vi "saveGlobalVar-2.vi"() -> ()   [LabVIEW 2019]
uses:
  GlobalVariable1.vi
panel:
  out "Waveform Chart":dbl(graph)
  in  "stop":bool
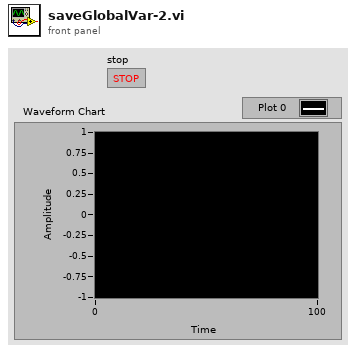
[diagram p1: front panel]
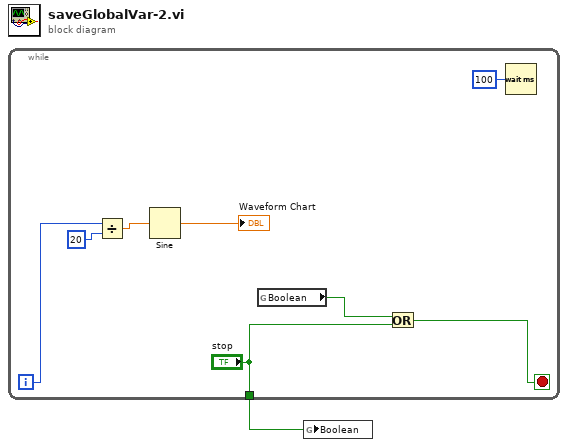
[diagram p0: block diagram]
diagram:
  n1 = while {
    tunnel: ["stop"] -> w1
    i -> [w9]
    stop <- w3 stop-if-true
    n2 = Divide(x=w9, y=20) -> (x/y=w7:dbl)
    n3 = Sine(x=w7) -> (sin(x)=→"Waveform Chart":dbl)
    n4 = global read "GlobalVariable1.vi" "Boolean"() -> (w4:bool)
    n5 = Or(x=w4, y="stop") -> (x .or. y?=w3:bool)
    n6 = Wait (ms)(milliseconds to wait=u32 100) -> ()  [unwired: 1 out]
  }
  n7 = global write "GlobalVariable1.vi" "Boolean"(w1) -> ()
